vi "Filter and Data Scaling backup (062609).vi"(0 "Offset Data":string[](array[string]), 5 "Slope Data":string[](array[string]), 7 "Filter Data":string[](array[string]), 9 "Vin":dbl[](array[numeric]), 11 "error in":errorcluster, 12 "Allow Zero?":string[](array[string])) -> (4 "Vout":string[](array[string]), 6 "Offset Data":string[](array[string]), 8 "ScaledOut":string[](array[string]), 10 "ScaledOut":dbl[](array[numeric]), 14 "Allow Zero?":string[](array[string]), 15 "error out":errorcluster)   [LabVIEW 2009]
uses:
  <vilib>/ptbypt/NI_PtbyPt.lvlib
panel:
  # "32-51= FM1 GPM Data Point 1-20"
  # "32-51= FM1 Data Point # 1-20"
  # "32-51 = FM1 K Factor 1-20"
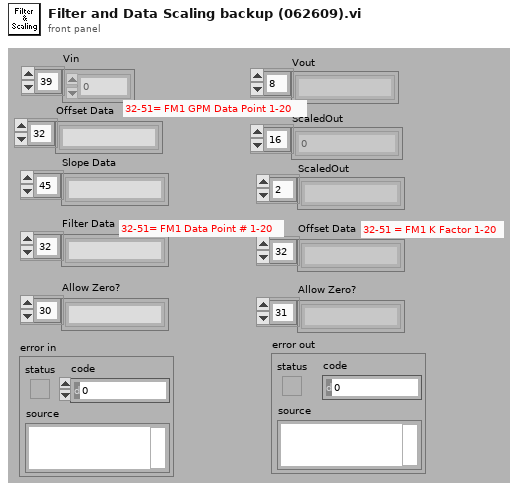
[diagram p1: front panel]
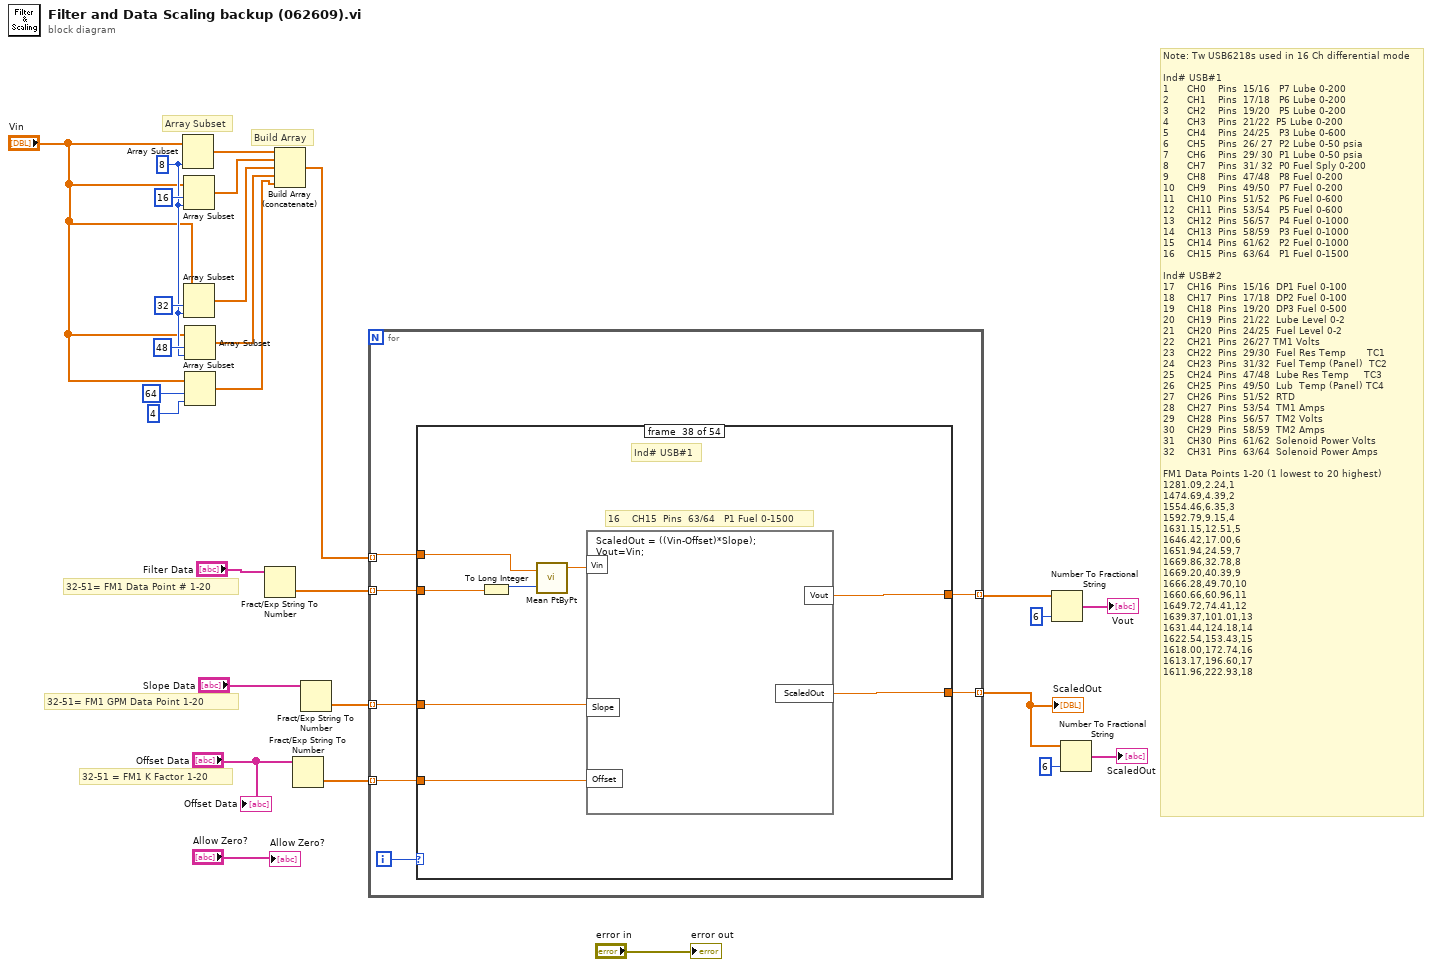
[diagram p0: block diagram]
diagram:
  w7 = 8 ("length")
  # "32-51 = FM1 K Factor 1-20"
  # "32-51= FM1 Data Point # 1-20"
  # "32-51= FM1 GPM Data Point 1-20"
  # "Array Subset"
  # "Build Array"
  # "Note: Tw USB6218s used in 16 Ch differential mode\n\nInd# USB#1\n1      CH0\t\t  Pins  15/16\t  P7 Lube 0-200\n2      CH1\t\t  Pins  17/18\t  P6 Lube 0-200\n3      CH2\t\t  Pins  19/20   P5 Lube 0-200\n4      CH3\t\t  Pins  21/22  P5 Lube 0-200\n5      CH4\t   Pins  24/25\t  P3 Lube 0-600\n6      CH5\t\t  Pins  26/\t27\t P2 Lube 0-50 psia\n7      CH6\t   Pins  29/\t30\t P1 Lube 0-50 psia\n8      CH7\t  \tPins  31/ 32\t P0 Fuel Sply 0-200  \n9      CH8\t  \tPins  47/48\t  P8 Fuel 0-200   \n10    CH9\t\t  Pins  49/50\t  P7 Fuel 0-200   \n11    CH10\t\tPins  51/52\t  P6 Fuel 0-600   \n12    CH11\t\tPins  53/54\t  P5 Fuel 0-600   \n13    CH12\t\tPins  56/57\t  P4 Fuel 0-1000 \n14    CH13\t\tPins  58/59\t  P3 Fuel 0-1000 \n15    CH14\t\tPins  61/62 \t P2 Fuel 0-1000  \n16    CH15\t\tPins  63/64 \t P1 Fuel 0-1500 \n\nInd# USB#2\n17    CH16\t\tPins  15/16\t DP1 Fuel 0-100 \n18    CH17\t\tPins  17/18\t DP2 Fuel 0-100\n19    CH18\t\tPins  19/20  DP3 Fuel 0-500 \n20    CH19\t Pins  21/22\t Lube Level 0-2 \n21    CH20\t\tPins  24/25\t Fuel Level 0-2 \n22    CH21\t\tPins  26/27\tTM1 Volts  \n23    CH22\t Pins  29/30  Fuel Res Temp       TC1\n24    CH23\t\tPins  31/32\t Fuel Temp (Panel)  TC2 \n25    CH24\t\tPins \t47/48\t Lube Res Temp     TC3 \n26    CH25\t\tPins  49/50\t Lub  Temp (Panel) TC4 \n27    CH26\t\tPins  51/52\t RTD \n28    CH27\t\tPins  53/54\t TM1 Amps \n29    CH28\t\tPins  56/57\t TM2 Volts\n30    CH29\t\tPins  58/59\t TM2 Amps \n31    CH30\t\tPins  61/62  Solenoid Power Volts \n32    CH31\t\tPins  63/64  Solenoid Power Amps\n\nFM1 Data Points 1-20 (1 lowest to 20 highest)\n1281.09,2.24,1\n1474.69,4.39,2\n1554.46,6.35,3\n1592.79,9.15,4\n1631.15,12.51,5\n1646.42,17.00,6\n1651.94,24.59,7\n1669.86,32.78,8\n1669.20,40.39,9\n1666.28,49.70,10\n1660.66,60.96,11\n1649.72,74.41,12\n1639.37,101.01,13\n1631.44,124.18,14\n1622.54,153.43,15\n1618.00,172.74,16\n1613.17,196.60,17\n1611.96,222.93,18"
  n1 = Array Subset(array="Vin", length=w7) -> (w12:dbl[])  [unwired: 1 in]
  n2 = Array Subset(array="Vin", index=16, length=w7) -> (w11:dbl[])
  n3 = Array Subset(array="Vin", index=32, length=w7) -> (w9:dbl[])
  n4 = Array Subset(array="Vin", index=48, length=w7) -> (w10:dbl[])
  n5 = Array Subset(array="Vin", index=64, length=4 ("index")) -> (w2:dbl[])
  n6 = Fract/Exp String To Number(string="Filter Data") -> (number=w22:dbl[])  [unwired: 4 out]
  n7 = Build Array (concatenate)(w12, w11, w9, w10, w2) -> (w1:dbl[])
  n8 = Fract/Exp String To Number(string="Offset Data") -> (number=w23:dbl[])  [unwired: 4 out]
  n9 = Fract/Exp String To Number(string="Slope Data") -> (number=w24:dbl[])  [unwired: 4 out]
  n10 = for {
    tunnel: w24 -> [w33] mode=indexing
    tunnel: w23 -> [w32] mode=indexing
    tunnel: w22 -> [w34] mode=indexing
    tunnel: [w30] -> w6 mode=indexing
    tunnel: [w31] -> w15 mode=indexing
    tunnel: w1 -> [w28] mode=indexing
    i -> [w29]
    n11 = case shown="32" w29 {
      selector: w29 -> [_ _ _ _ _ _ _ _ _ _ _ _ _ _ _ _ _ _ _ _ _ _ _ _ w58 _ _ _ _ w100 _ _ _ _ _ _ _ _ _ _ _ _ _ _ _ _ _ _ _ _ _ _ _ _]
      tunnel: w28 -> [_ _ _ _ _ _ _ _ _ _ _ _ _ _ _ _ _ _ _ _ _ _ w43 w49 w63 w69 w77 w85 w93 w105 w111 w119 w127 w135 w143 w151 w159 w167 w175 w183 w191 w199 w207 w215 w223 w231 w239 w247 w255 w263 w271 w279 w287 w295]
      tunnel: w34 -> [_ _ _ _ _ _ _ _ _ _ _ _ _ _ _ _ _ _ _ _ _ _ w44 w50 w64 w70 w78 w86 w94 w106 w112 w120 w128 w136 w144 w152 w160 w168 w176 w184 w192 w200 w208 w216 w224 w232 w240 w248 w256 w264 w272 w280 w288 w296]
      tunnel: w33 -> [w35 w36 w37 w38 _ _ _ _ _ _ _ _ _ _ _ _ _ _ _ _ _ _ w42 w52 w62 w68 w76 w84 w92 w104 w110 w118 w126 w134 w142 w150 w158 w166 w174 w182 w190 w198 w206 w214 w222 w230 w238 w246 w254 w262 w270 w278 w286 w294]
      tunnel: w32 -> [_ _ _ _ _ _ _ _ _ _ _ _ _ _ _ _ _ _ _ _ _ _ w41 w51 w61 w67 w75 w83 w91 w103 w109 w117 w125 w133 w141 w149 w157 w165 w173 w181 w189 w197 w205 w213 w221 w229 w237 w245 w253 w261 w269 w277 w285 w293]
      tunnel: [_ _ _ _ _ _ _ _ _ _ _ _ _ _ _ _ _ _ _ _ _ _ w39 w48 w59 w65 w73 w81 w89 w101 w107 w115 w123 w131 w139 w147 w155 w163 w171 w179 w187 w195 w203 w211 w219 w227 w235 w243 w251 w259 w267 w275 w283 w291] -> w31
      tunnel: [w35 w36 w37 w38 _ _ _ _ _ _ _ _ _ _ _ _ _ _ _ _ _ _ w40 w47 w60 w66 w74 w82 w90 w102 w108 w116 w124 w132 w140 w148 w156 w164 w172 w180 w188 w196 w204 w212 w220 w228 w236 w244 w252 w260 w268 w276 w284 w292] -> w30
      frame #0 {
        # "FM1 Data Point"
        # "FM1 GPM"
        # "K factor"
        # "Flowmeter scale"
      }
      frame #1 {
        # "FM1 Data Point"
        # "FM1 GPM"
        # "K factor"
        # "Flowmeter scale"
      }
      frame #2 {
        # "FM1 Data Point"
        # "FM1 GPM"
        # "K factor"
        # "Flowmeter scale"
      }
      frame #3 {
        # "Flow meter scale"
      }
      frame #4 {
      }
      frame #5 {
      }
      frame #6 {
      }
      frame #7 {
      }
      frame #8 {
      }
      frame #9 {
      }
      frame #10 {
      }
      frame #11 {
      }
      frame #12 {
      }
      frame #13 {
      }
      frame #14 {
      }
      frame #15 {
      }
      frame #16 {
      }
      frame #17 {
      }
      frame #18 {
      }
      frame #19 {
      }
      frame #20 {
      }
      frame #21 {
      }
      frame #22 {
        # "Ind# USB#1"
        # "1      CH0\t\t  Pins  15/16\t  P7 Lube 0-200"
        n12 = To Long Integer(number=w44) -> (32bit integer=w46:i32)
        n13 = call <vilib>:"Mean PtByPt.vi"("x"=w43, "sample length"=w46) -> ("mean"=w45:dbl)  [unwired: 1 in, 2 out]
        n14 = formula code="ScaledOut = ((Vin-Offset)*Slope);\nVout=Vin;"("Vin"=w45, "Slope"=w42, "Offset"=w41) -> ("ScaledOut"=w40:dbl, "Vout"=w39:dbl)
      }
      frame #23 {
        # "Ind# USB#1"
        # "2      CH1\t\t  Pins  17/18\t  P6 Lube 0-200"
        n15 = To Long Integer(number=w50) -> (32bit integer=w54:i32)
        n16 = call <vilib>:"Mean PtByPt.vi"("x"=w49, "sample length"=w54) -> ("mean"=w53:dbl)  [unwired: 1 in, 2 out]
        n17 = formula code="ScaledOut = ((Vin-Offset)*Slope);\nVout=Vin;"("Vin"=w53, "Slope"=w52, "Offset"=w51) -> ("ScaledOut"=w47:dbl, "Vout"=w48:dbl)
      }
      frame #24 {
        # "Ind# USB#1"
        # "3      CH2\t\t  Pins  19/20   P5 Lube 0-200"
        n18 = To Long Integer(number=w64) -> (32bit integer=w57:i32)
        n19 = Equal To 0?(x=w58) -> (x = 0?=w56:bool)
        n20 = call <vilib>:"Mean PtByPt.vi"("x"=w63, "sample length"=w57, "initialize"=w56) -> ("mean"=w55:dbl)  [unwired: 2 out]
        n21 = formula code="ScaledOut = ((Vin-Offset)*Slope);\nVout=Vin;"("Vin"=w55, "Slope"=w62, "Offset"=w61) -> ("ScaledOut"=w60:dbl, "Vout"=w59:dbl)
      }
      frame #25 {
        # "Ind# USB#1"
        # "4      CH3\t\t  Pins  21/22  P5 Lube 0-200"
        n22 = To Long Integer(number=w70) -> (32bit integer=w72:i32)
        n23 = call <vilib>:"Mean PtByPt.vi"("x"=w69, "sample length"=w72) -> ("mean"=w71:dbl)  [unwired: 1 in, 2 out]
        n24 = formula code="ScaledOut = ((Vin-Offset)*Slope);\nVout=Vin;"("Vin"=w71, "Slope"=w68, "Offset"=w67) -> ("ScaledOut"=w66:dbl, "Vout"=w65:dbl)
      }
      frame #26 {
        # "Ind# USB#1"
        # "5      CH4\t   Pins  24/25\t  P3 Lube 0-600"
        n25 = To Long Integer(number=w78) -> (32bit integer=w80:i32)
        n26 = call <vilib>:"Mean PtByPt.vi"("x"=w77, "sample length"=w80) -> ("mean"=w79:dbl)  [unwired: 1 in, 2 out]
        n27 = formula code="ScaledOut = ((Vin-Offset)*Slope);\nVout=Vin;"("Vin"=w79, "Slope"=w76, "Offset"=w75) -> ("ScaledOut"=w74:dbl, "Vout"=w73:dbl)
      }
      frame #27 {
        # "6      CH5\t\t  Pins  26/\t27\t P2 Lube 0-50 psia"
        # "Ind# USB#1"
        n28 = To Long Integer(number=w86) -> (32bit integer=w88:i32)
        n29 = call <vilib>:"Mean PtByPt.vi"("x"=w85, "sample length"=w88) -> ("mean"=w87:dbl)  [unwired: 1 in, 2 out]
        n30 = formula code="ScaledOut = ((Vin-Offset)*Slope);\nVout=Vin;"("Vin"=w87, "Slope"=w84, "Offset"=w83) -> ("ScaledOut"=w82:dbl, "Vout"=w81:dbl)
      }
      frame #28 {
        # "7      CH6\t   Pins  29/\t30\t P1 Lube 0-50 psia"
        # "Ind# USB#1"
        n31 = To Long Integer(number=w94) -> (32bit integer=w96:i32)
        n32 = call <vilib>:"Mean PtByPt.vi"("x"=w93, "sample length"=w96) -> ("mean"=w95:dbl)  [unwired: 1 in, 2 out]
        n33 = formula code="ScaledOut = ((Vin-Offset)*Slope);\nVout=Vin;"("Vin"=w95, "Slope"=w92, "Offset"=w91) -> ("ScaledOut"=w90:dbl, "Vout"=w89:dbl)
      }
      frame #29 {
        # "8      CH7\t  \tPins  31/ 32\t P0 Fuel Sply 0-200"
        # "Ind# USB#1"
        n34 = To Long Integer(number=w106) -> (32bit integer=w98:i32)
        n35 = Equal To 0?(x=w100) -> (x = 0?=w99:bool)
        n36 = call <vilib>:"Mean PtByPt.vi"("x"=w105, "sample length"=w98, "initialize"=w99) -> ("mean"=w97:dbl)  [unwired: 2 out]
        n37 = formula code="ScaledOut = ((Vin-Offset)*Slope);\nVout=Vin;"("Vin"=w97, "Slope"=w104, "Offset"=w103) -> ("ScaledOut"=w102:dbl, "Vout"=w101:dbl)
      }
      frame #30 {
        # "9      CH8\t  \tPins  47/48\t  P8 Fuel 0-200"
        # "Ind# USB#1"
        n38 = To Long Integer(number=w112) -> (32bit integer=w114:i32)
        n39 = call <vilib>:"Mean PtByPt.vi"("x"=w111, "sample length"=w114) -> ("mean"=w113:dbl)  [unwired: 1 in, 2 out]
        n40 = formula code="ScaledOut = ((Vin-Offset)*Slope);\nVout=Vin;"("Vin"=w113, "Slope"=w110, "Offset"=w109) -> ("ScaledOut"=w108:dbl, "Vout"=w107:dbl)
      }
      frame #31 {
        # "10    CH9\t\t  Pins  49/50\t  P7 Fuel 0-200"
        # "Ind# USB#1"
        n41 = To Long Integer(number=w120) -> (32bit integer=w122:i32)
        n42 = call <vilib>:"Mean PtByPt.vi"("x"=w119, "sample length"=w122) -> ("mean"=w121:dbl)  [unwired: 1 in, 2 out]
        n43 = formula code="ScaledOut = ((Vin-Offset)*Slope);\nVout=Vin;"("Vin"=w121, "Slope"=w118, "Offset"=w117) -> ("ScaledOut"=w116:dbl, "Vout"=w115:dbl)
      }
      frame #32 {
        # "11    CH10\t\tPins  51/52\t  P6 Fuel 0-600"
        # "Ind# USB#1"
        n44 = To Long Integer(number=w128) -> (32bit integer=w130:i32)
        n45 = call <vilib>:"Mean PtByPt.vi"("x"=w127, "sample length"=w130) -> ("mean"=w129:dbl)  [unwired: 1 in, 2 out]
        n46 = formula code="ScaledOut = ((Vin-Offset)*Slope);\nVout=Vin;"("Vin"=w129, "Slope"=w126, "Offset"=w125) -> ("ScaledOut"=w124:dbl, "Vout"=w123:dbl)
      }
      frame #33 {
        # "12    CH11\t\tPins  53/54\t  P5 Fuel 0-600"
        # "Ind# USB#1"
        n47 = To Long Integer(number=w136) -> (32bit integer=w138:i32)
        n48 = call <vilib>:"Mean PtByPt.vi"("x"=w135, "sample length"=w138) -> ("mean"=w137:dbl)  [unwired: 1 in, 2 out]
        n49 = formula code="ScaledOut = ((Vin-Offset)*Slope);\nVout=Vin;"("Vin"=w137, "Slope"=w134, "Offset"=w133) -> ("ScaledOut"=w132:dbl, "Vout"=w131:dbl)
      }
      frame #34 {
        # "13    CH12\t\tPins  56/57\t  P4 Fuel 0-1000"
        # "Ind# USB#1"
        n50 = To Long Integer(number=w144) -> (32bit integer=w146:i32)
        n51 = call <vilib>:"Mean PtByPt.vi"("x"=w143, "sample length"=w146) -> ("mean"=w145:dbl)  [unwired: 1 in, 2 out]
        n52 = formula code="ScaledOut = ((Vin-Offset)*Slope);\nVout=Vin;"("Vin"=w145, "Slope"=w142, "Offset"=w141) -> ("ScaledOut"=w140:dbl, "Vout"=w139:dbl)
      }
      frame #35 {
        # "14    CH13\t\tPins  58/59\t  P3 Fuel 0-1000"
        # "Ind# USB#1"
        n53 = To Long Integer(number=w152) -> (32bit integer=w154:i32)
        n54 = call <vilib>:"Mean PtByPt.vi"("x"=w151, "sample length"=w154) -> ("mean"=w153:dbl)  [unwired: 1 in, 2 out]
        n55 = formula code="ScaledOut = ((Vin-Offset)*Slope);\nVout=Vin;"("Vin"=w153, "Slope"=w150, "Offset"=w149) -> ("ScaledOut"=w148:dbl, "Vout"=w147:dbl)
      }
      frame #36 {
        # "15    CH14\t\tPins  61/62 \t P2 Fuel 0-1000"
        # "Ind# USB#1"
        n56 = To Long Integer(number=w160) -> (32bit integer=w162:i32)
        n57 = call <vilib>:"Mean PtByPt.vi"("x"=w159, "sample length"=w162) -> ("mean"=w161:dbl)  [unwired: 1 in, 2 out]
        n58 = formula code="ScaledOut = ((Vin-Offset)*Slope);\nVout=Vin;"("Vin"=w161, "Slope"=w158, "Offset"=w157) -> ("ScaledOut"=w156:dbl, "Vout"=w155:dbl)
      }
      frame #37 {
        # "16    CH15\t\tPins  63/64 \t P1 Fuel 0-1500"
        # "Ind# USB#1"
        n59 = To Long Integer(number=w168) -> (32bit integer=w170:i32)
        n60 = call <vilib>:"Mean PtByPt.vi"("x"=w167, "sample length"=w170) -> ("mean"=w169:dbl)  [unwired: 1 in, 2 out]
        n61 = formula code="ScaledOut = ((Vin-Offset)*Slope);\nVout=Vin;"("Vin"=w169, "Slope"=w166, "Offset"=w165) -> ("ScaledOut"=w164:dbl, "Vout"=w163:dbl)
      }
      frame #38 {
        # "17    CH16\t\tPins  15/16\t DP1 Fuel 0-100"
        # "Ind# USB#1"
        n62 = To Long Integer(number=w176) -> (32bit integer=w178:i32)
        n63 = call <vilib>:"Mean PtByPt.vi"("x"=w175, "sample length"=w178) -> ("mean"=w177:dbl)  [unwired: 1 in, 2 out]
        n64 = formula code="ScaledOut = ((Vin-Offset)*Slope);\nVout=Vin;"("Vin"=w177, "Slope"=w174, "Offset"=w173) -> ("ScaledOut"=w172:dbl, "Vout"=w171:dbl)
      }
      frame #39 {
        # "18    CH17\t\tPins  17/18\t DP2 Fuel 0-100"
        # "Ind# USB#2"
        n65 = To Long Integer(number=w184) -> (32bit integer=w186:i32)
        n66 = call <vilib>:"Mean PtByPt.vi"("x"=w183, "sample length"=w186) -> ("mean"=w185:dbl)  [unwired: 1 in, 2 out]
        n67 = formula code="ScaledOut = ((Vin-Offset)*Slope);\nVout=Vin;"("Vin"=w185, "Slope"=w182, "Offset"=w181) -> ("ScaledOut"=w180:dbl, "Vout"=w179:dbl)
      }
      frame #40 {
        # "19    CH18\t\tPins  19/20  DP3 Fuel 0-500"
        # "Ind# USB#2"
        n68 = To Long Integer(number=w192) -> (32bit integer=w194:i32)
        n69 = call <vilib>:"Mean PtByPt.vi"("x"=w191, "sample length"=w194) -> ("mean"=w193:dbl)  [unwired: 1 in, 2 out]
        n70 = formula code="ScaledOut = ((Vin-Offset)*Slope);\nVout=Vin;"("Vin"=w193, "Slope"=w190, "Offset"=w189) -> ("ScaledOut"=w188:dbl, "Vout"=w187:dbl)
      }
      frame #41 {
        # "20    CH19\t Pins  21/22\t Lube Level 0-2"
        # "Ind# USB#2"
        n71 = To Long Integer(number=w200) -> (32bit integer=w202:i32)
        n72 = call <vilib>:"Mean PtByPt.vi"("x"=w199, "sample length"=w202) -> ("mean"=w201:dbl)  [unwired: 1 in, 2 out]
        n73 = formula code="ScaledOut = ((Vin-Offset)*Slope);\nVout=Vin;"("Vin"=w201, "Slope"=w198, "Offset"=w197) -> ("ScaledOut"=w196:dbl, "Vout"=w195:dbl)
      }
      frame #42 {
        # "21    CH20\t\tPins  24/25\t Fuel Level 0-2"
        # "Ind# USB#2"
        n74 = To Long Integer(number=w208) -> (32bit integer=w210:i32)
        n75 = call <vilib>:"Mean PtByPt.vi"("x"=w207, "sample length"=w210) -> ("mean"=w209:dbl)  [unwired: 1 in, 2 out]
        n76 = formula code="ScaledOut = ((Vin-Offset)*Slope);\nVout=Vin;"("Vin"=w209, "Slope"=w206, "Offset"=w205) -> ("ScaledOut"=w204:dbl, "Vout"=w203:dbl)
      }
      frame #43 {
        # "22    CH21\t\tPins  26/27\tTM1 Volts"
        # "Ind# USB#2"
        n77 = To Long Integer(number=w216) -> (32bit integer=w218:i32)
        n78 = call <vilib>:"Mean PtByPt.vi"("x"=w215, "sample length"=w218) -> ("mean"=w217:dbl)  [unwired: 1 in, 2 out]
        n79 = formula code="ScaledOut = ((Vin-Offset)*Slope);\nVout=Vin;"("Vin"=w217, "Slope"=w214, "Offset"=w213) -> ("ScaledOut"=w212:dbl, "Vout"=w211:dbl)
      }
      frame #44 {
        # "23    CH22\t Pins  29/30  Fuel Res Temp       TC1"
        # "Ind# USB#2"
        n80 = To Long Integer(number=w224) -> (32bit integer=w226:i32)
        n81 = call <vilib>:"Mean PtByPt.vi"("x"=w223, "sample length"=w226) -> ("mean"=w225:dbl)  [unwired: 1 in, 2 out]
        n82 = formula code="ScaledOut = ((Vin-Offset)*Slope);\nVout=Vin;"("Vin"=w225, "Slope"=w222, "Offset"=w221) -> ("ScaledOut"=w220:dbl, "Vout"=w219:dbl)
      }
      frame #45 {
        # "24    CH23\t\tPins  31/32\t Fuel Temp (Panel)  TC2"
        # "Ind# USB#2"
        n83 = To Long Integer(number=w232) -> (32bit integer=w234:i32)
        n84 = call <vilib>:"Mean PtByPt.vi"("x"=w231, "sample length"=w234) -> ("mean"=w233:dbl)  [unwired: 1 in, 2 out]
        n85 = formula code="ScaledOut = ((Vin-Offset)*Slope);\nVout=Vin;"("Vin"=w233, "Slope"=w230, "Offset"=w229) -> ("ScaledOut"=w228:dbl, "Vout"=w227:dbl)
      }
      frame #46 {
        # "25    CH24\t\tPins \t47/48\t Lube Res Temp     TC3"
        # "Ind# USB#2"
        n86 = To Long Integer(number=w240) -> (32bit integer=w242:i32)
        n87 = call <vilib>:"Mean PtByPt.vi"("x"=w239, "sample length"=w242) -> ("mean"=w241:dbl)  [unwired: 1 in, 2 out]
        n88 = formula code="ScaledOut = ((Vin-Offset)*Slope);\nVout=Vin;"("Vin"=w241, "Slope"=w238, "Offset"=w237) -> ("ScaledOut"=w236:dbl, "Vout"=w235:dbl)
      }
      frame #47 {
        # "26    CH25\t\tPins  49/50\t Lub  Temp (Panel) TC4"
        # "Ind# USB#2"
        n89 = To Long Integer(number=w248) -> (32bit integer=w250:i32)
        n90 = call <vilib>:"Mean PtByPt.vi"("x"=w247, "sample length"=w250) -> ("mean"=w249:dbl)  [unwired: 1 in, 2 out]
        n91 = formula code="ScaledOut = ((Vin-Offset)*Slope);\nVout=Vin;"("Vin"=w249, "Slope"=w246, "Offset"=w245) -> ("ScaledOut"=w244:dbl, "Vout"=w243:dbl)
      }
      frame #48 {
        # "27    CH26\t\tPins  51/52\t RTD"
        # "Ind# USB#2"
        n92 = To Long Integer(number=w256) -> (32bit integer=w258:i32)
        n93 = call <vilib>:"Mean PtByPt.vi"("x"=w255, "sample length"=w258) -> ("mean"=w257:dbl)  [unwired: 1 in, 2 out]
        n94 = formula code="ScaledOut = ((Vin-Offset)*Slope);\nVout=Vin;"("Vin"=w257, "Slope"=w254, "Offset"=w253) -> ("ScaledOut"=w252:dbl, "Vout"=w251:dbl)
      }
      frame #49 {
        # "28    CH27\t\tPins  53/54\t TM1 Amps"
        # "Ind# USB#2"
        n95 = To Long Integer(number=w264) -> (32bit integer=w266:i32)
        n96 = call <vilib>:"Mean PtByPt.vi"("x"=w263, "sample length"=w266) -> ("mean"=w265:dbl)  [unwired: 1 in, 2 out]
        n97 = formula code="ScaledOut = ((Vin-Offset)*Slope);\nVout=Vin;"("Vin"=w265, "Slope"=w262, "Offset"=w261) -> ("ScaledOut"=w260:dbl, "Vout"=w259:dbl)
      }
      frame #50 {
        # "29    CH28\t\tPins  56/57\t TM2 Volts"
        # "Ind# USB#2"
        n98 = To Long Integer(number=w272) -> (32bit integer=w274:i32)
        n99 = call <vilib>:"Mean PtByPt.vi"("x"=w271, "sample length"=w274) -> ("mean"=w273:dbl)  [unwired: 1 in, 2 out]
        n100 = formula code="ScaledOut = ((Vin-Offset)*Slope);\nVout=Vin;"("Vin"=w273, "Slope"=w270, "Offset"=w269) -> ("ScaledOut"=w268:dbl, "Vout"=w267:dbl)
      }
      frame #51 {
        # "30    CH29\t\tPins  58/59\t TM2 Amps"
        # "Ind# USB#2"
        n101 = To Long Integer(number=w280) -> (32bit integer=w282:i32)
        n102 = call <vilib>:"Mean PtByPt.vi"("x"=w279, "sample length"=w282) -> ("mean"=w281:dbl)  [unwired: 1 in, 2 out]
        n103 = formula code="ScaledOut = ((Vin-Offset)*Slope);\nVout=Vin;"("Vin"=w281, "Slope"=w278, "Offset"=w277) -> ("ScaledOut"=w276:dbl, "Vout"=w275:dbl)
      }
      frame #52 {
        # "31    CH30\t\tPins  61/62  Solenoid Power Volts"
        # "Ind# USB#2"
        n104 = To Long Integer(number=w288) -> (32bit integer=w290:i32)
        n105 = call <vilib>:"Mean PtByPt.vi"("x"=w287, "sample length"=w290) -> ("mean"=w289:dbl)  [unwired: 1 in, 2 out]
        n106 = formula code="ScaledOut = ((Vin-Offset)*Slope);\nVout=Vin;"("Vin"=w289, "Slope"=w286, "Offset"=w285) -> ("ScaledOut"=w284:dbl, "Vout"=w283:dbl)
      }
      frame #53 {
        # "32    CH31\t\tPins  63/64  Solenoid Power Amps"
        # "Ind# USB#2"
        n107 = To Long Integer(number=w296) -> (32bit integer=w298:i32)
        n108 = call <vilib>:"Mean PtByPt.vi"("x"=w295, "sample length"=w298) -> ("mean"=w297:dbl)  [unwired: 1 in, 2 out]
        n109 = formula code="ScaledOut = ((Vin-Offset)*Slope);\nVout=Vin;"("Vin"=w297, "Slope"=w294, "Offset"=w293) -> ("ScaledOut"=w292:dbl, "Vout"=w291:dbl)
      }
    }
  }
  "ScaledOut" <- w6
  n110 = Number To Fractional String(number=w15, precision (6)=i16 6) -> (F-format string=→"Vout":string[])  [unwired: 2 out]
  n111 = Number To Fractional String(number=w6, precision (6)=i16 6) -> (F-format string=→"ScaledOut":string[])  [unwired: 2 out]
  "Allow Zero?" <- "Allow Zero?"
  "Offset Data" <- "Offset Data"
  "error out" <- "error in"
